vi "To-simple-string.vi"(8 "error in (no error)":errorcluster, 11 "Move-Absolute in":refnum<class "Move-Absolute.lvclass">) -> (0 "error out":errorcluster, 2 "Action string":string, 3 "Move-Absolute out":refnum<class "Move-Absolute.lvclass">)   [LabVIEW 2013, in "PowderDeposition.lvlib" / "Move-Absolute.lvclass"]
uses:
  Move-Absolute.lvclass
  Move-Absolute.lvclass/Move-Absolute.ctl
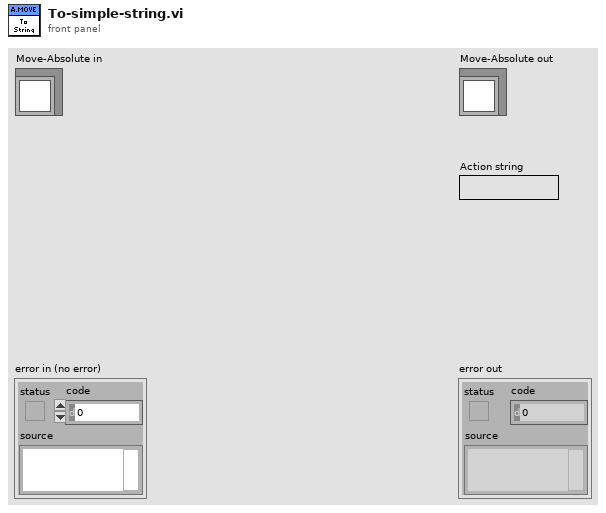
[diagram p1: front panel]
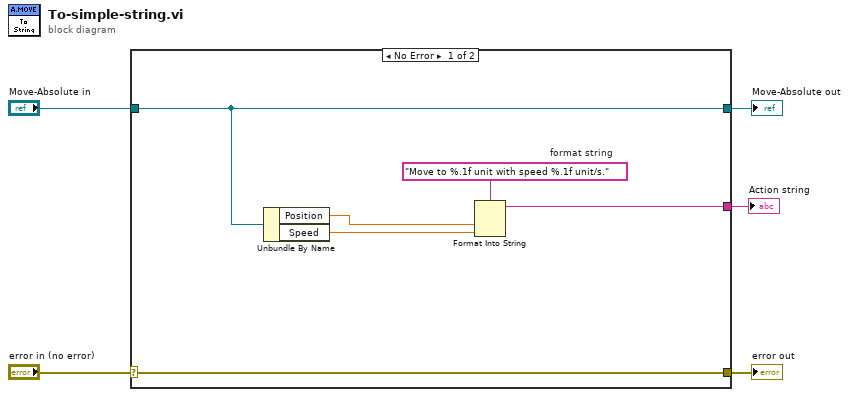
[diagram p0: block diagram]
diagram:
  n1 = case shown="No Error" "error in (no error)" {
    selector: "error in (no error)" -> [w11 w13]
    tunnel: [w11 w13] -> w4
    tunnel: [w8 w12] -> w2
    tunnel: "Move-Absolute in" -> [w8 w12]
    tunnel: [w9 _] -> w1
    frame No Error {
      w10 = "Move to %.1f unit with speed %.1f unit/s."  # format string
      n2 = Unbundle By Name(w8) -> ("Position"=w7:dbl, "Speed"=w6:dbl)
      n3 = Format Into String(format string=w10, w7, w6) -> (resulting string=w9:string)  [unwired: 2 in, 1 out]
    }
    frame Error {
    }
  }
  "error out" <- w4
  "Move-Absolute out" <- w2
  "Action string" <- w1
